vi "test derivatives.vi"() -> ()   [LabVIEW 2017]
uses:
  typedefs/magnet location fit result.ctl
panel:
  out "dBz":dbl[](array[numeric])
  out "dBy":dbl[](array[numeric])
  out "dBz numeric":dbl[](array[numeric])
  out "dBy numeric":dbl[](array[numeric])
  out "dBx numeric":dbl[](array[numeric])
  out "dBx":dbl[](array[numeric])
  out "Bx (uT)":dbl
  in  "magnet location params":T1={"x magnet"=0.0, "y magnet"=0.0, "z magnet"=75.0, "Br*V (T*mm^3)"=500.0, "theta - moment angle to z-axis"=0.0, "phi - moment angle to x-axis"=0.0}
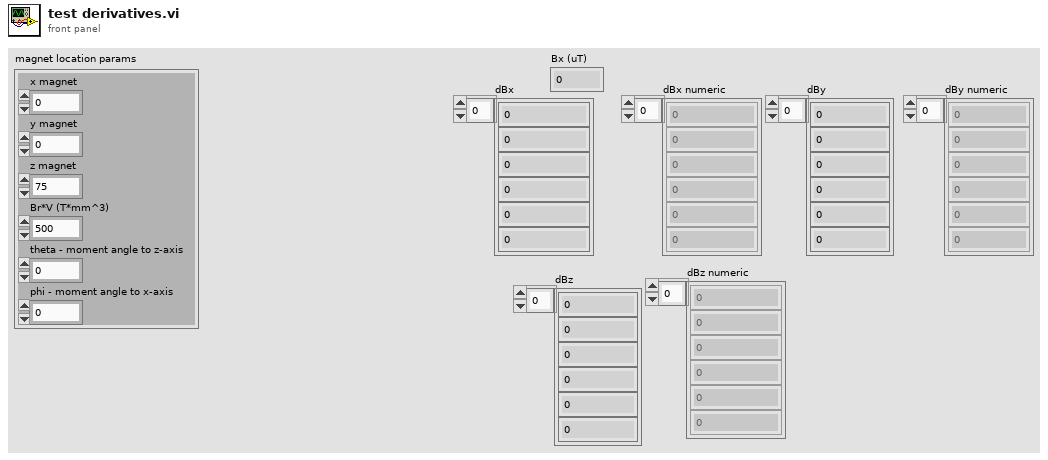
[diagram p1: front panel]
types:
  T1 = typedef "magnet location fit result.ctl" = cluster{"x magnet":dbl, "y magnet":dbl, "z magnet":dbl, "Br*V (T*mm^3)":dbl, "theta - moment angle to z-axis":dbl, "phi - moment angle to x-axis":dbl}
  T2 = cluster{"magnet location params[0]":dbl, "magnet location params[1]":dbl, "magnet location params[2]":dbl, "magnet location params[3]":dbl, "magnet location params[4]":dbl, "magnet location params[5]":dbl}
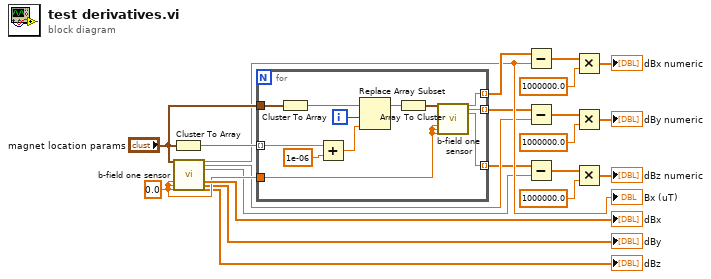
[diagram p0: block diagram]
diagram:
  w18 = 0.0 ("x sensor")
  n1 = Cluster To Array(cluster="magnet location params") -> (array=w20:dbl[])
  n2 = call "b-field one sensor.vi"("magnet location params"="magnet location params", "x sensor"=w18, "y sensor"=w18, "z sensor"=w18) -> ("Bx (uT)"=w16:dbl, "By (uT)"=w9:dbl, "Bz (uT)"=w4:dbl, "dBx"=→"dBx":dbl[], "dBy"=→"dBy":dbl[], "dBz"=→"dBz":dbl[])  [unwired: 18 in]
  "Bx (uT)" <- w16
  n3 = for {
    tunnel: w20 -> [w30] mode=indexing
    tunnel: "magnet location params" -> [w33]
    tunnel: w18 -> [w26]
    tunnel: [w25] -> w17 mode=indexing
    tunnel: [w24] -> w10 mode=indexing
    tunnel: [w23] -> w5 mode=indexing
    i -> [w31]
    n4 = Cluster To Array(cluster=w33) -> (array=w32:dbl[])
    n5 = Add(x=w30, y=1e-06) -> (x+y=w22:dbl)
    n6 = Replace Array Subset(array=w32, new element=w22, index=w31) -> (w28:dbl[])
    n7 = Array To Cluster(array=w28) -> (cluster=w27:T2)
    n8 = call "b-field one sensor.vi"("magnet location params"=w27, "x sensor"=w26, "y sensor"=w26, "z sensor"=w26) -> ("Bx (uT)"=w25:dbl, "By (uT)"=w24:dbl, "Bz (uT)"=w23:dbl)  [unwired: 18 in, 3 out]
  }
  n9 = Subtract(x=w17, y=w16) -> (x-y=w15:dbl[])
  n10 = Subtract(x=w10, y=w9) -> (x-y=w12:dbl[])
  n11 = Subtract(x=w5, y=w4) -> (x-y=w7:dbl[])
  n12 = Multiply(x=w15, y=1000000.0) -> (x*y=→"dBx numeric":dbl[])
  n13 = Multiply(x=w12, y=1000000.0) -> (x*y=→"dBy numeric":dbl[])
  n14 = Multiply(x=w7, y=1000000.0) -> (x*y=→"dBz numeric":dbl[])
